vi "Create Evaluations.vi"(8 "error in (no error)":errorcluster, 11 "Skyworks - 2G PVT in":refnum<class "Skyworks - 2G PVT.lvclass">) -> (0 "error out":errorcluster, 1 "Evaluations Out":T1[](array[typedef]) {"Low Limit" format="%#_13g"; "SI Scaling" items=["femto"=-15, "pico"=-12, "nano"=-9, "micro"=-6, "milli"=-3, "percent"=-2, ""=0, "kilo"=3, "mega"=6, "giga"=9, "tera"=12]}, 3 "Skyworks - 2G PVT out":refnum<class "Skyworks - 2G PVT.lvclass">)   [LabVIEW 2016, in "Skyworks - 2G PVT.lvlib" / "Skyworks - 2G PVT.lvclass"]
uses:
  Skyworks - 2G PVT.lvclass
  C:/Sequence Automation/Plugins/Measurement Interface.lvlibp/Measurement Interface.lvclass
  C:/Sequence Automation/Plugins/Measurements/Skyworks - PVT.lvlibp/Skyworks - PVT.lvclass
  Plugins/TestStand API Tools (TSAT).lvlibp/Evaluation Actions/Includes/Controls/TSAT Evaluation.ctl
  Plugins/TestStand API Tools (TSAT).lvlibp/Evaluation Actions/Includes/Controls/TSAT Eval SI Unit Scaling.ctl
  Plugins/TestStand API Tools (TSAT).lvlibp/Evaluation Actions/Includes/Controls/TSAT Evaluation Type.ctl
  Plugins/Measurement Interface.lvlibp/Private Methods/Measurement Name/Read Measurement Name.vi
  Plugins/SeqAuto Evaluations.lvlibp/Skyworks/2G_PVT/Skyworks_2G_PVT.lvclass
  Plugins/TestStand API Tools (TSAT).lvlibp/Evaluation Actions/TSAT Evaluation Actions.lvlib
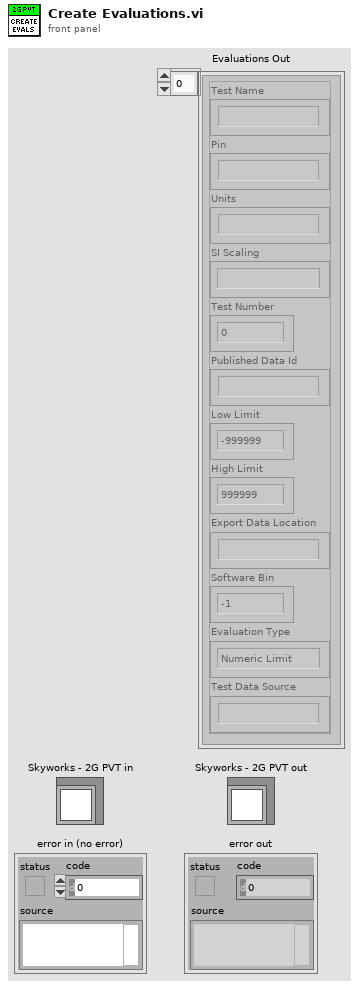
[diagram p1: front panel]
types:
  T1 = typedef "TestStand API Tools (TSAT).lvlibp/TSAT Evaluation Actions.lvlib/TSAT Evaluation.ctl" = cluster{"Test Name":string, "Pin":string, "Units":string, "SI Scaling":T2, "Test Number":i32, "Published Data Id":string, "Low Limit":dbl, "High Limit":dbl, "Export Data Location":string, "Software Bin":i64, "Evaluation Type":T3, "Test Data Source":string}
  T2 = typedef "TestStand API Tools (TSAT).lvlibp/TSAT Evaluation Actions.lvlib/TSAT Eval SI Unit Scaling.ctl" = i16
  T3 = typedef "TestStand API Tools (TSAT).lvlibp/TSAT Evaluation Actions.lvlib/TSAT Evaluation Type.ctl" = enum16{"Numeric Limit", "Pass/Fail", "None"}
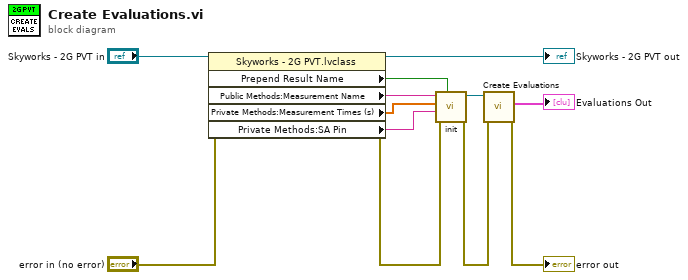
[diagram p0: block diagram]
diagram:
  n1 = property class="Skyworks - 2G PVT.lvclass"(reference="Skyworks - 2G PVT in", error in="error in (no error)") -> (reference out=→"Skyworks - 2G PVT out":refnum<class "Skyworks - 2G PVT.lvclass">, error out=w6:errorcluster, "Prepend Result Name"=w11:bool, "Public Methods:Measurement Name"=w10:string, "Private Methods:Measurement Times (s)"=w8:dbl[], "Private Methods:SA Pin"=w7:string)
  n2 = call "init.vi"("Prepend Result Name"=w11, "error in (no error)"=w6, "SA Pin"=w7, "Measurement Times (s)"=w8, "Measurement Name"=w10) -> ("error out"=w3:errorcluster, "Skyworks_2G_PVT out"=w12:refnum<class "Skyworks_2G_PVT.lvclass">)  [unwired: 5 in]
  n3 = call-dynamic "Create Evaluations.vi"("error in (no error)"=w3, "IEvaluation in"=w12) -> ("error out"=→"error out":errorcluster, "Evaluations Out"=→"Evaluations Out":T1[])  [unwired: 7 in, 1 out]
